vi "test2_xq3.vi"() -> ()   [LabVIEW 2018]
uses:
  <vilib>/imath/engines/lvmath/Plug In/_Char/NIMS_CH_character datatype.ctl
  <vilib>/imath/engines/lvmath/Plug In/_Char/NIMS_CH_Character RV to String.vi
  <vilib>/imath/engines/lvmath2/RunTimeEngine/BuiltInFunctions/random/NIMS_random.vi
  <vilib>/imathl/engines/lvmath/Functions/Error Handling/Create Error.vi
  <vilib>/imath/engines/lvmath2/RunTimeEngine/BuiltInFunctions/fir_win/NIMS_fir_win(I32,V,Str,V,Str).vi
  <vilib>/imath/engines/lvmath2/RunTimeEngine/ErrorHandling/NIMS_Create Error From Enums.vi
  <vilib>/imath/engines/lvmath2/RunTimeEngine/BuiltInFunctions/fft/NIMS_fft(GV).vi
  <instcachedir>/0/NIMS_fft(GV)_4C6467FC22F84E4BA42517A07EF978B0.lvgen/NIMS_fft(GV)_4C6467FC22F84E4BA42517A07EF978B0_000.vi
  <vilib>/imath/engines/lvmath2/RunTimeEngine/ErrorHandling/NIMS_Error From Error Code.vi
  <vilib>/imath/engines/lvmath2/RunTimeEngine/BuiltInFunctions/crosscorr/NIMS_crosscorr(GM,Str).vi
  <instcachedir>/0/NIMS_crosscorr(GM,Str)_B40E69E1A515490ABE9B33FB59F56A52.lvgen/NIMS_crosscorr(GM,Str)_B40E69E1A515490ABE9B33FB59F56A52_000.vi
  <vilib>/imath/engines/lvmath2/RunTimeEngine/BuiltInFunctions/fft/NIMS_fft(GM).vi
  <instcachedir>/0/NIMS_fft(GM)_4D6538E03936427980510B9710B4978C.lvgen/NIMS_fft(GM)_4D6538E03936427980510B9710B4978C_000.vi
  <vilib>/imath/engines/lvmath2/RunTimeEngine/ArithmeticOperatorToken/NIMS_ArithmeticOperator_power(S).vi
  <instcachedir>/0/NIMS_ArithmeticOperator_power(S)_E7916602C36D4BDA819D832F61F93EE1.lvgen/NIMS_ArithmeticOperator_power(S)_E7916602C36D4BDA819D832F61F93EE1_012.vi
  <vilib>/imath/engines/lvmath2/RunTimeEngine/BuiltInFunctions/abs/NIMS_abs(signed).vi
  <instcachedir>/0/NIMS_abs(signed)_C4FCB8E6058B49B797C7C8D53CA5F6EC.lvgen/NIMS_abs(signed)_C4FCB8E6058B49B797C7C8D53CA5F6EC_003.vi
  <instcachedir>/0/NIMS_abs(signed)_C4FCB8E6058B49B797C7C8D53CA5F6EC.lvgen/NIMS_abs(signed)_C4FCB8E6058B49B797C7C8D53CA5F6EC_006.vi
  <vilib>/imath/engines/lvmath2/RunTimeEngine/ArithmeticOperatorToken/NIMS_ArithmeticOperator_times.vi
  <instcachedir>/0/NIMS_ArithmeticOperator_times_D7E4A7A4AD2C4409A0CE309D2741A5B4.lvgen/NIMS_ArithmeticOperator_times_D7E4A7A4AD2C4409A0CE309D2741A5B4_007.vi
  <vilib>/imath/engines/lvmath2/RunTimeEngine/BuiltInFunctions/ifft/NIMS_ifft(CM).vi
  <vilib>/imath/engines/lvmath2/RunTimeEngine/BuiltInFunctions/fftshift/NIMS_fftshift(GM).vi
  <instcachedir>/0/NIMS_fftshift(GM)_854644D58B904BE68890FF38C728418A.lvgen/NIMS_fftshift(GM)_854644D58B904BE68890FF38C728418A_003.vi
  <vilib>/imath/engines/lvmath2/RunTimeEngine/RangeToken/NIMS_Range.vi
  <instcachedir>/0/NIMS_Range_846134F467D14A349F7C6CCEF459CDB2.lvgen/NIMS_Range_846134F467D14A349F7C6CCEF459CDB2_000.vi
  <vilib>/imath/engines/lvmath2/RunTimeEngine/NodeEndStatement/NIMS_NodeEndStatement_Get Vector.vi
  <instcachedir>/0/NIMS_NodeEndStatement_Get Vector_329D0992E87F49F089135171B7FC9327.lvgen/NIMS_NodeEndStatement_Get Vector_329D0992E87F49F089135171B7FC9327_003.vi
  <instcachedir>/0/NIMS_NodeEndStatement_Get Vector_329D0992E87F49F089135171B7FC9327.lvgen/NIMS_NodeEndStatement_Get Vector_329D0992E87F49F089135171B7FC9327_001.vi
  <vilib>/imath/engines/lvmath/Functions/Error Handling/MergeErrorsWrapper.vi
  <vilib>/imath/engines/lvmath2/RunTimeEngine/NodeEndStatement/NIMS_NodeEndStatement_Output.vi
  <instcachedir>/0/NIMS_NodeEndStatement_Output_53EC0D466D134D7ABD903AC30B43404B.lvgen/NIMS_NodeEndStatement_Output_53EC0D466D134D7ABD903AC30B43404B_005.vi
  <instcachedir>/0/NIMS_NodeEndStatement_Output_53EC0D466D134D7ABD903AC30B43404B.lvgen/NIMS_NodeEndStatement_Output_53EC0D466D134D7ABD903AC30B43404B_002.vi
  <instcachedir>/0/NIMS_NodeEndStatement_Output_53EC0D466D134D7ABD903AC30B43404B.lvgen/NIMS_NodeEndStatement_Output_53EC0D466D134D7ABD903AC30B43404B_000.vi
  <vilib>/imath/engines/lvmath2/RunTimeEngine/ErrorHandling/NIMS_Finalize Error.vi
panel:
  out "HW":cluster{"BIN":dbl[], "N":dbl[]}(graph)
  out "Ryy":cluster{"BIN":dbl[], "N":dbl[]}(graph)
  out "Syy":cluster{"BIN":dbl[], "N":dbl[]}(graph)
  out "HW^2":cluster{"BIN":dbl[], "N":dbl[]}(graph)
  out "RXX":dbl[][](graph)
  out "ht":dbl[](graph)
  out "xt":dbl[][](graph)
  out "Sxx":cluster{"BIN":dbl[], "N":dbl[]}(graph)
  in  "N":dbl=500.0
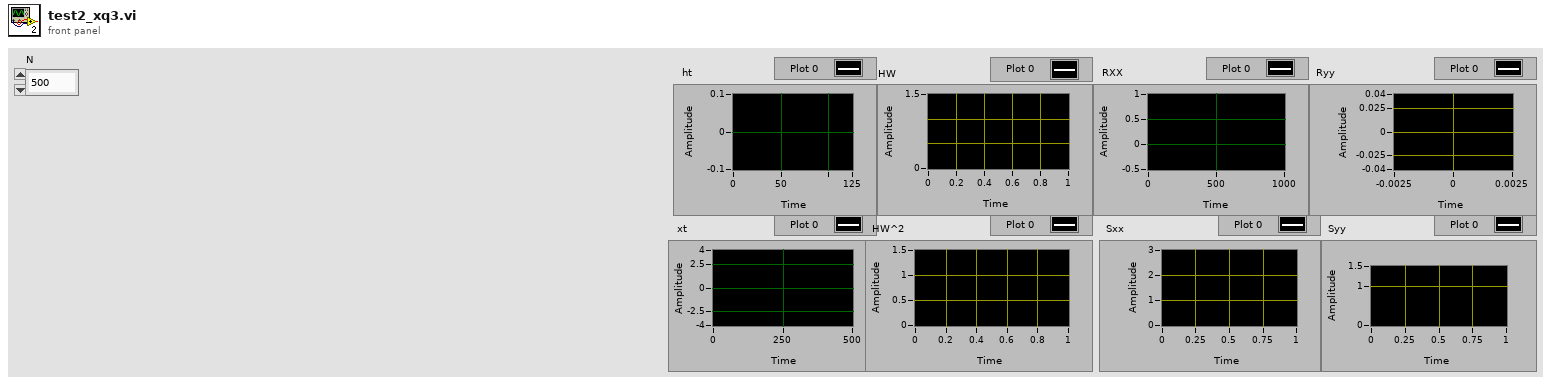
[diagram p1: front panel]
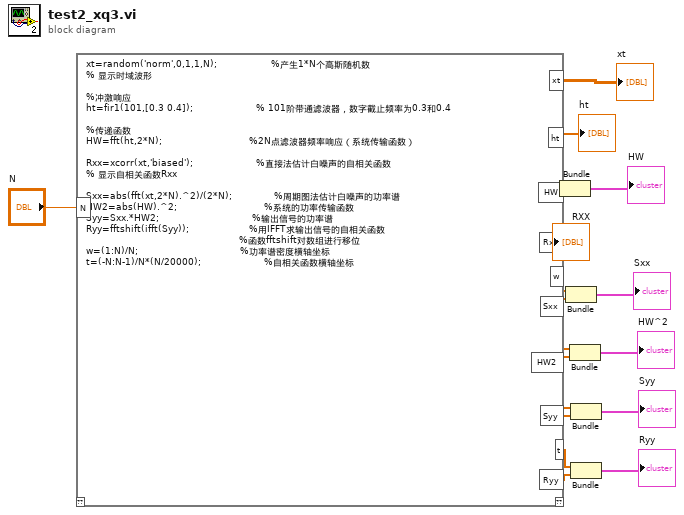
[diagram p0: block diagram]
diagram:
  n1 = mathscript code="xt=random('norm',0,1,1,N);                  %产生1*N个高斯随机数\n% 显示时域波形\n\n%冲激响应\nht=fir1(101,[0.3 0.4]);                     % 101阶带通滤波器，数字截止频率为0.3和0.4\n\n%传递函数\nHW=fft(ht,2*N);                             %2N点滤波器频率响应（系统传输函数）\n\nRxx=xcorr(xt,'biased');                     %直接法估计白噪声的自相关函数\n% 显示自相关函数Rxx\n\nSxx=abs(fft(xt,2*N).^2)/(2*N);              %周期图法估计白噪声的功率谱\nHW2=abs(HW).^2;                             %系统的功率传输函数\nSyy=Sxx.*HW2;                               %输出信号的功率谱\nRyy=fftshift(ifft(Syy));                    %用IFFT求输出信号的自相关函数\n                                                   %函数fftshift对数组进行移位\nw=(1:N)/N;                                  %功率谱密度横轴坐标\nt=(-N:N-1)/N*(N/20000);                     %自相关函数横轴坐标"("N"="N") -> ("xt"=→"xt":dbl[][], "ht"=→"ht":dbl[], "HW"=w2:cdb[], "Rxx"=→"RXX":dbl[][], "w"=w1:dbl[], "Sxx"=w11:dbl[], "HW2"=w9:dbl[], "Syy"=w7:dbl[], "t"=w5:dbl[], "Ryy"=w4:dbl[])  [unwired: 1 in, 1 out]
  n2 = Bundle("w"=w1, "HW"=w2) -> (→"HW":cluster{"w":dbl[], "HW":cdb[]})  [unwired: 1 in]
  n3 = Bundle("w"=w1, "Sxx"=w11) -> (→"Sxx":cluster{"w":dbl[], "Sxx":dbl[]})  [unwired: 1 in]
  n4 = Bundle("w"=w1, "HW2"=w9) -> (→"HW^2":cluster{"w":dbl[], "HW2":dbl[]})  [unwired: 1 in]
  n5 = Bundle("w"=w1, "Syy"=w7) -> (→"Syy":cluster{"w":dbl[], "Syy":dbl[]})  [unwired: 1 in]
  n6 = Bundle("t"=w5, "Ryy"=w4) -> (→"Ryy":cluster{"t":dbl[], "Ryy":dbl[]})  [unwired: 1 in]
